vi "Arm Distance to Angle Convert.vi"(10 "Angle In":dbl format="%#_13g", 11 "Distance In":dbl format="%#_13g") -> (2 "Distance Out":dbl, 3 "Angle Out":dbl)   [LabVIEW 2018]
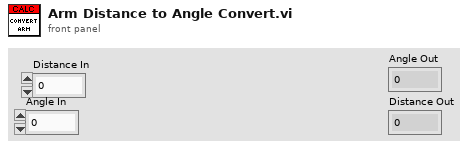
[diagram p1: front panel]
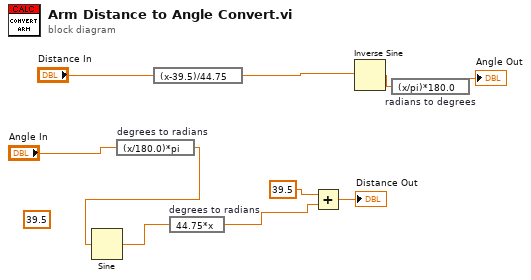
[diagram p0: block diagram]
diagram:
  (unwired) 39.5
  n1 = expression code="(x/180.0)*pi" "degrees to radians"("Angle In") -> (w3:dbl)
  n2 = Sine(x=w3) -> (sin(x)=w5:dbl)
  n3 = expression code="(x-39.5)/44.75"("Distance In") -> (w2:dbl)
  n4 = expression code="44.75*x" "degrees to radians"(w5) -> (w6:dbl)
  n5 = Add(x=39.5, y=w6) -> (x+y=→"Distance Out":dbl)
  n6 = Inverse Sine(1:w2) -> (0:w9:dbl)
  n7 = expression code="(x/pi)*180.0" "radians to degrees"(w9) -> (→"Angle Out":dbl)
